vi "Read data from PXImc_NonRegion.vi"(8 "error in (no error)":errorcluster, 11 "RT Data Cluster in":T1 {"StatusRefs" format="%.0x"; "ReceiveRefs"."Data Reference" format="%.0x"; "SendRefs"."Data Reference" format="%.0x"}) -> (0 "error out":errorcluster, 3 "RT Data Cluster out":T1 {"StatusRefs" format="%.0x"; "ReceiveRefs"."Data Reference" format="%.0x"; "SendRefs"."Data Reference" format="%.0x"})   [LabVIEW 2016, in "PXImc Engine.lvlib"]
uses:
  PXImc Engine.lvlib
  RT Data Cluster.ctl
  Shared/Compiled Data.ctl
  <vilib>/NI Veristand/Custom Device API/Block Data Reference.ctl
  <vilib>/NI Veristand/Custom Device API/Data Reference.ctl
  <vilib>/NI Veristand/Custom Device API/Global Data Refs.vi
  <vilib>/pximc/Read (DBL).vi
  <vilib>/NI Veristand/Custom Device API/Custom Device API.lvlib
  <vilib>/pximc/nipximc.lvlib
  <resource>/objmgr/pximc.rc
  Shared/PXImc Shared.lvlib
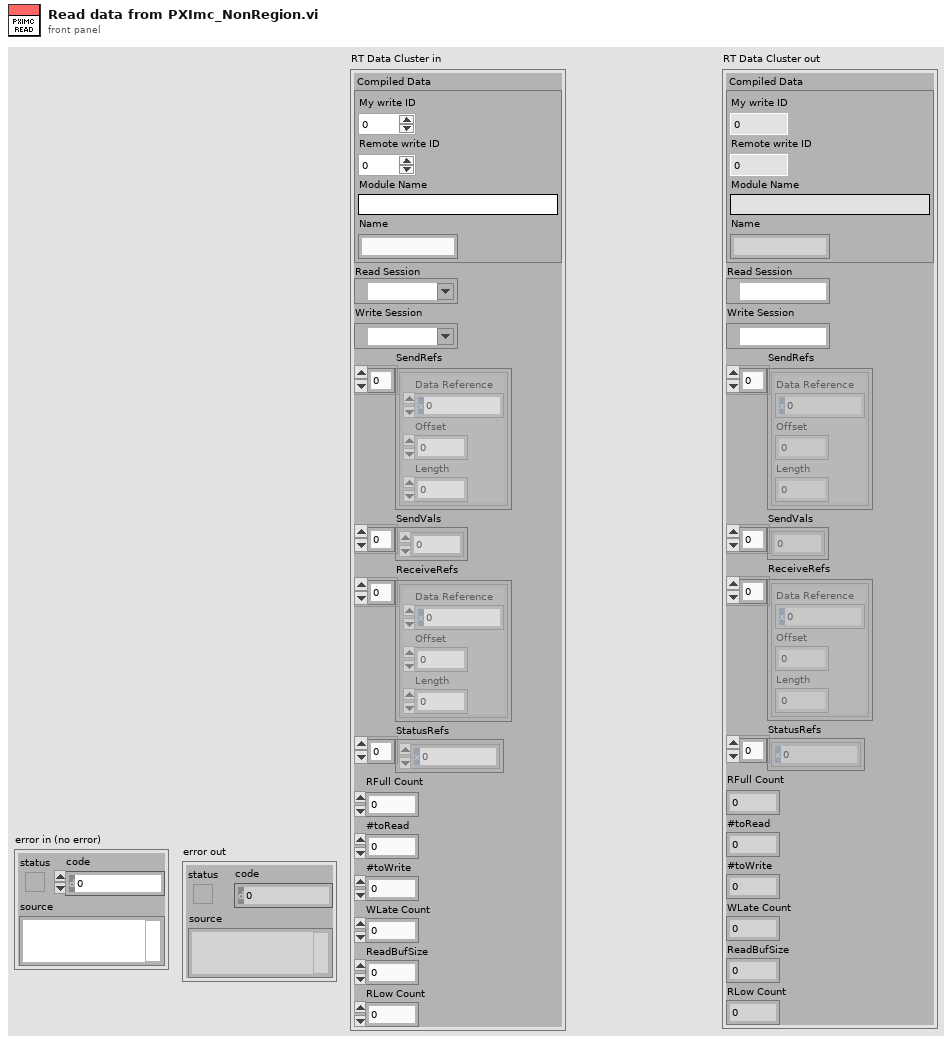
[diagram p1: front panel]
types:
  T1 = typedef "PXImc Engine.lvlib/RT Data Cluster.ctl" = cluster{"Compiled Data":T2, "Read Session":refnum<k21>, "Write Session":refnum<k21>, "SendRefs":T3[], "SendVals":dbl[], "ReceiveRefs":T3[], "StatusRefs":T4[], "RFull Count":dbl, "#toRead":i32, "#toWrite":i32, "WLate Count":dbl, "ReadBufSize":i32, "RLow Count":dbl}
  T2 = typedef "PXImc Shared.lvlib/Compiled Data.ctl" = cluster{"My write ID":u16, "Remote write ID":u16, "Module Name":string, "Name":string}
  T3 = typedef "Custom Device API.lvlib/Block Data Reference.ctl" = cluster{"Data Reference":T4, "Offset":u64, "Length":u64}
  T4 = typedef "Custom Device API.lvlib/Data Reference.ctl" = i32
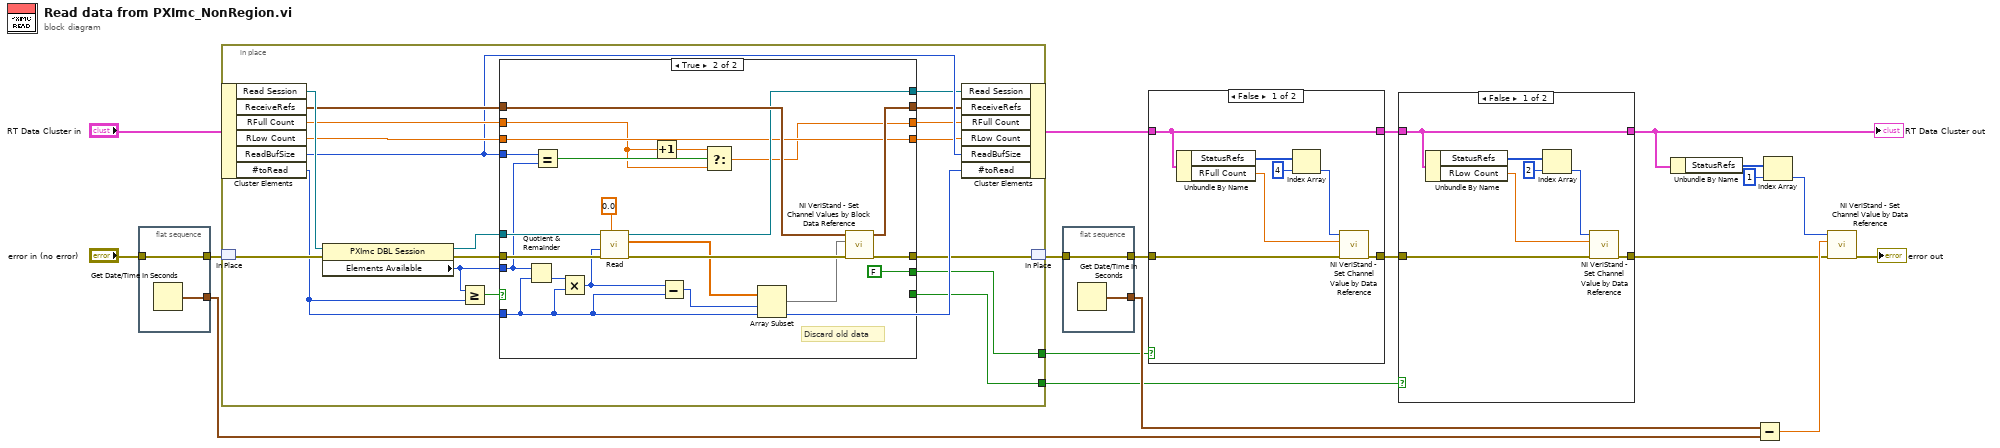
[diagram p0: block diagram]
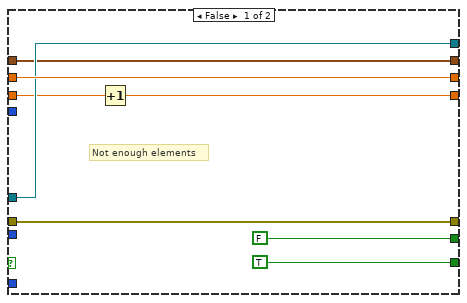
[diagram p4: hidden frame]
diagram:
  n1 = flat-sequence {
    tunnel: [w21] -> w19
    tunnel: "error in (no error)" -> [w21]
    tunnel: [w20] -> w12
    frame #0 {
      n2 = Get Date/Time In Seconds() -> (seconds since 1Jan1904=w20:timestamp)
    }
  }
  n3 = in-place {
    in-place-border: [w23] -> w6
    in-place-border: [w22] -> w1
    n4 = in-place-cluster #1("RT Data Cluster in") -> ("Read Session"=w38:refnum<k21>, "ReceiveRefs"=w37:T3[], "RFull Count"=w36:dbl, "RLow Count"=w35:dbl, "ReadBufSize"=w34:i32, "#toRead"=w30:i32)
    n5 = in-place-match #2(w19) -> (w39:errorcluster)
    n6 = property class="PXImc DBL Session"(reference=w38, error in=w39) -> (reference out=w33:refnum<k21>, error out=w32:errorcluster, "Elements Available"=w31:u64)
    n7 = Greater Or Equal?(x=w31, y=w30) -> (x >= y?=w29:bool)
    n8 = case shown="True" w29 {
      tunnel: [w45 w64] -> w28
      tunnel: w36 -> [w47 w49]
      tunnel: [w47 w48] -> w26
      tunnel: [w46 w69] -> w24
      tunnel: w37 -> [w44 w66]
      tunnel: [w44 w65] -> w27
      tunnel: w32 -> [w46 w68]
      tunnel: w33 -> [w45 w67]
      tunnel: w30 -> [_ w55]
      tunnel: w34 -> [_ w61]
      tunnel: w31 -> [_ w58]
      tunnel: [FALSE FALSE] -> w23
      tunnel: w35 -> [w42 w62]
      tunnel: [w41 w62] -> w25
      tunnel: [TRUE _] -> w22
      frame False {
        # "Not enough elements"
        n9 = Increment(x=w42) -> (x+1=w41:dbl)
      }
      frame True {
        # "Discard old data"
        n10 = Quotient & Remainder(x=w58, y=w55) -> (floor(x/y)=w57:u64)  [unwired: 1 out]
        n11 = Equal?(x=w61, y=w58) -> (x = y?=w50:bool)
        n12 = Multiply(x=w57, y=w55) -> (x*y=w56:u64)
        n13 = call-poly <vilib>:"Read.vi"("timeout in seconds (5)"=0.0, "error in (no error)"=w68, "number of elements"=w56, "session in"=w67) -> ("error out"=w59:errorcluster, "data"=w53:dbl[], "session out"=w64:refnum<k21>)  [unwired: 5 in]
        n14 = Increment(x=w49) -> (x+1=w51:dbl)
        n15 = Subtract(x=w56, y=w55) -> (x-y=w54:u64)
        n16 = Select(t=w51, s=w50, f=w49) -> (s? t:f=w48:dbl)
        n17 = Array Subset(array=w53, index=w54, length=w55) -> (w52:dbl[])
        n18 = call <vilib>:"NI VeriStand - Set Channel Values by Block Data Reference.vi"("error in (no error)"=w59, "Values Array in"=w52, "Block Data Ref"=w66) -> ("error out"=w69:errorcluster, "Block Data Ref dup"=w65:T3[])  [unwired: 6 in, 1 out]
      }
    }
    n19 = in-place-cluster #1("Read Session"=w28, "ReceiveRefs"=w27, "RFull Count"=w26, "RLow Count"=w25, "ReadBufSize"=w34, "#toRead"=w30) -> (w14:T1)
    n20 = in-place-match #2(w24) -> (w16:errorcluster)
  }
  n21 = flat-sequence {
    tunnel: [w71] -> w15
    tunnel: w16 -> [w71]
    tunnel: [w70] -> w13
    frame #0 {
      n22 = Get Date/Time In Seconds() -> (seconds since 1Jan1904=w70:timestamp)
    }
  }
  n23 = case shown="False" w6 {
    tunnel: w15 -> [w78 w80]
    tunnel: w14 -> [w72 w79]
    tunnel: [w73 w80] -> w4
    tunnel: [w72 w79] -> w5
    frame False {
      n24 = Unbundle By Name(w72) -> ("StatusRefs"=w77:T4[], "RFull Count"=w74:dbl)
      n25 = Index Array(array=w77, index=4) -> (element=w75:T4)
      n26 = call <vilib>:"NI VeriStand - Set Channel Value by Data Reference.vi"("error in (no error)"=w78, "Value"=w74, "Data Reference in"=w75) -> ("error out"=w73:errorcluster)  [unwired: 8 in]
    }
    frame True {
    }
  }
  n27 = case shown="False" w1 {
    tunnel: w4 -> [w87 w89]
    tunnel: w5 -> [w81 w88]
    tunnel: [w82 w89] -> w2
    tunnel: [w81 w88] -> w3
    frame False {
      n28 = Unbundle By Name(w81) -> ("StatusRefs"=w86:T4[], "RLow Count"=w83:dbl)
      n29 = Index Array(array=w86, index=2) -> (element=w84:T4)
      n30 = call <vilib>:"NI VeriStand - Set Channel Value by Data Reference.vi"("error in (no error)"=w87, "Value"=w83, "Data Reference in"=w84) -> ("error out"=w82:errorcluster)  [unwired: 8 in]
    }
    frame True {
    }
  }
  "RT Data Cluster out" <- w3
  n31 = Unbundle By Name(w3) -> ("StatusRefs"=w11:T4[])
  n32 = Subtract(x=w13, y=w12) -> (x-y=w9:dbl)
  n33 = Index Array(array=w11, index=1) -> (element=w10:T4)
  n34 = call <vilib>:"NI VeriStand - Set Channel Value by Data Reference.vi"("error in (no error)"=w2, "Value"=w9, "Data Reference in"=w10) -> ("error out"=→"error out":errorcluster)  [unwired: 8 in]
